vi "threshold_stop(SubVI).vi"(9 "Stop threshold":dbl, 10 "Stop flashing below thresh":bool, 11 "dup path":path) -> (2 "Curr threshold":dbl, 3 "Boolean":bool)   [LabVIEW 2013]
uses:
  <vilib>/Utility/file.llb/Read From Spreadsheet File (DBL).vi
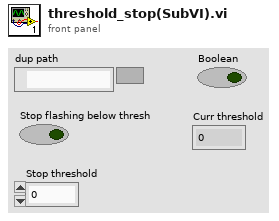
[diagram p1: front panel]
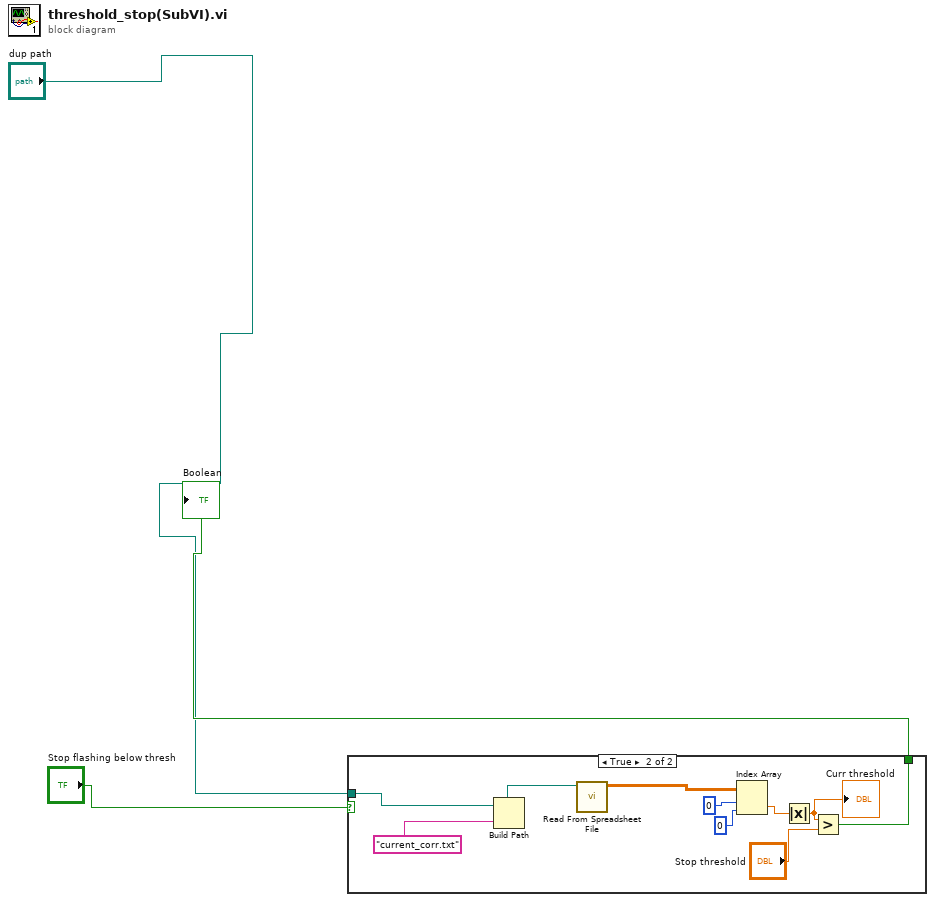
[diagram p0: block diagram]
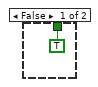
[diagram p2: hidden frame]
diagram:
  n1 = case shown="True" "Stop flashing below thresh" {
    tunnel: "dup path" -> [_ w14]
    tunnel: [TRUE w7] -> w3
    frame False {
    }
    frame True {
      n2 = Build Path(base path=w14, name or relative path="current_corr.txt") -> (appended path=w12:path)
      n3 = call-poly <vilib>:"Read From Spreadsheet File.vi"("file path (dialog if empty)"=w12) -> ("all rows"=w11:dbl[][])  [unwired: 6 in, 4 out]
      n4 = Index Array(array=w11, index (row)=0, index (col)=0 ("disabled index (col)")) -> (element=w6:dbl)
      n5 = Absolute Value(x=w6) -> (abs(x)=w5:dbl)
      "Curr threshold" <- w5
      n6 = Greater?(x=w5, y="Stop threshold") -> (0:w7:bool)
    }
  }
  "Boolean" <- w3
